vi "Polynomial Coefficients to Formula String.vi"(2 "Polynomial Coefficients":dbl[](array[numeric])) -> (7 "formula":string)   [LabVIEW 2021, in "Strings.lvlib"]
uses:
  Strings/Strings.lvlib
  74c6fc1e-1eae-41b4-a9e4-39dbf93ca976.vi
  74c6fc1e-1eae-41b4-a9e4-39dbf93ca976.vi/539bd7ec-d9e8-460f-a56d-a449b4a86a5e.vi
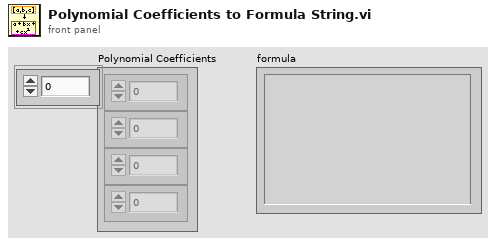
[diagram p1: front panel]
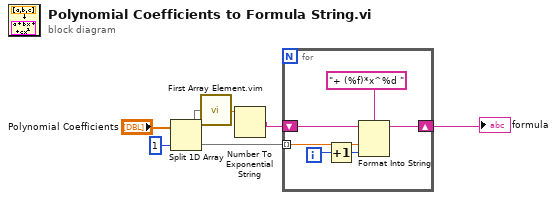
[diagram p0: block diagram]
diagram:
  n1 = Split 1D Array(array="Polynomial Coefficients", index=1) -> (first subarray=w3:dbl[], second subarray=w5:dbl[])
  n2 = call "First Array Element.vim"("Array"=w3) -> ("First Element"=w2:dbl)  [unwired: 8 in]
  n3 = Number To Exponential String(number=w2) -> (E-format string=w1:string)  [unwired: 3 in]
  n4 = for {
    shift-right: [w11] -> w6
    shift-left: w1 -> [w13]
    tunnel: w5 -> [w12] mode=indexing
    i -> [w9]
    n5 = Increment(x=w9) -> (x+1=w8:i32)
    n6 = Format Into String(format string="+ (%f)*x^%d ", initial string=w13, w12, w8) -> (resulting string=w11:string)  [unwired: 1 in, 1 out]
  }
  "formula" <- w6
